vi "Parse All Elements.vi"(8 "error in":errorcluster, 11 "Node in":refnum<k20>) -> (0 "error out":errorcluster, 1 "Properties out":refnum<class "Property.lvclass">[](array[class]), 2 "Channel Data":T1, 3 "Node out":refnum<k20>)   [LabVIEW 2024, in "Parser.lvlib" / "Channel.lvclass"]
uses:
  Channel.lvclass
  Property/Property.lvclass
  <vilib>/xml/Close Reference(Node).vi
  Channel.lvclass/Channel.ctl
  <resource>/objmgr/DOMUserDefRef.rc
  <vilib>/xml/NI_XML.lvlib
  Parser.lvlib
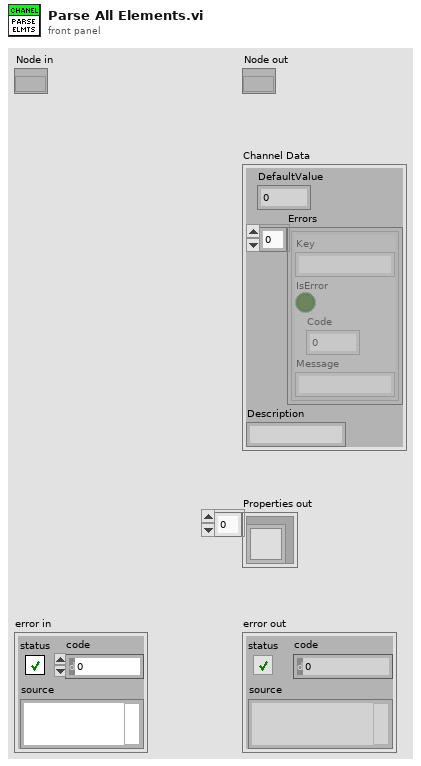
[diagram p1: front panel]
types:
  T1 = cluster{"DefaultValue":dbl, "Errors":cluster{"Key":string, "IsError":bool, "Code":u32, "Message":string}[], "Description":string}
  T2 = cluster{"Key":string, "IsError":bool, "Code":u32, "Message":string}[]
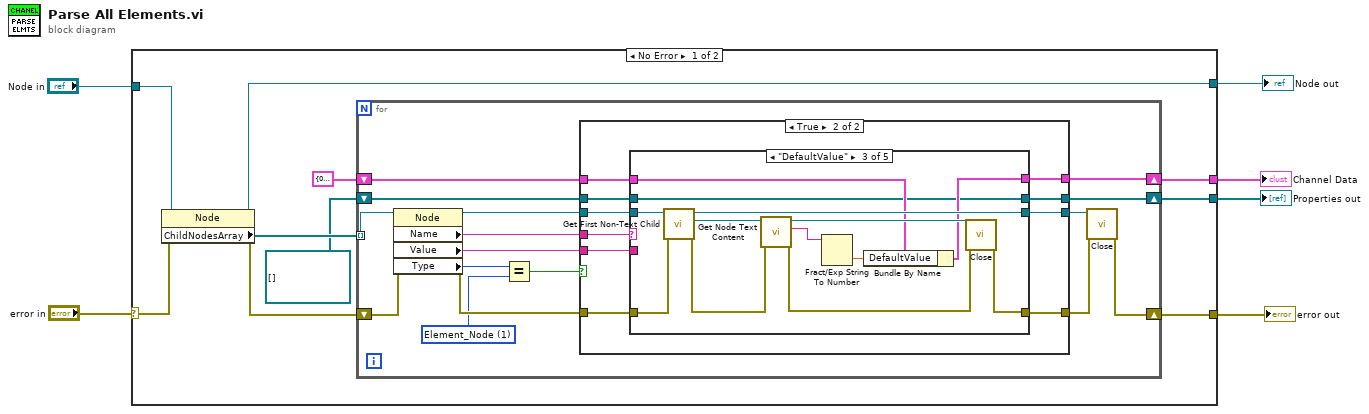
[diagram p0: block diagram]
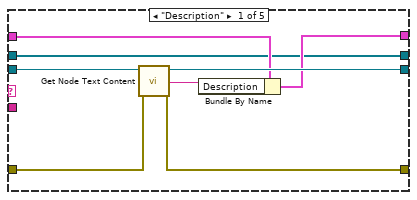
[diagram p3: hidden frame]
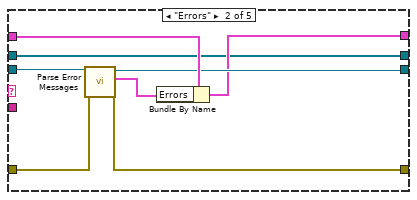
[diagram p4: hidden frame]
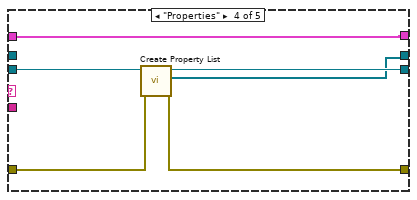
[diagram p5: hidden frame]
diagram:
  n1 = case shown="No Error" "error in" {
    selector: "error in" -> [w14 w87]
    tunnel: [w15 w87] -> w6
    tunnel: "Node in" -> [w13 w86]
    tunnel: [w11 _] -> w3
    tunnel: [w8 _] -> w2
    tunnel: [w7 w86] -> w1
    frame No Error {
      n2 = property class="Node"(reference=w13, error in=w14) -> (reference out=w7:refnum<k20>, error out=w16:errorcluster, "ChildNodesArray"=w10:refnum<k20>[])
      n3 = for {
        tunnel: w10 -> [w17] mode=indexing
        shift-right: [w31] -> w15
        shift-left: w16 -> [w32]
        shift-right: [w20] -> w11
        shift-left: T1 {"DefaultValue"=0.0, "Errors"=[], "Description"=""} ("Cluster of class private data") -> [w21]
        shift-right: [w18] -> w8
        shift-left: refnum<class "Property.lvclass">[] [] ("Properties") -> [w19]
        w24 = 1 items=["Element_Node"=1, "Attribute_Node"=2, "Text_Node"=3, "CDATASection_Node"=4, "EntityReference_Node"=5, "Entity_Node"=6, "ProcessingInstruction_Node"=7, "Comment_Node"=8, "Document_Node"=9, "DocumentType_Node"=10, "DocumentFragment_Node"=11, "Notation_Node"=12] ("Node Type")
        n4 = property on="Property Node" class="Node"(reference=w17, error in=w32) -> (reference out=w27:refnum<k20>, error out=w30:errorcluster, "Name"=w28:string, "Value"=w26:string, "Type"=w22:i32)
        n5 = Equal?(x=w22, y=w24) -> (x = y?=w23:bool)
        n6 = case shown="True" w23 {
          tunnel: w28 -> [_ w44]
          tunnel: w27 -> [w35 w43]
          tunnel: w26 -> [_ w42]
          tunnel: [w35 w41] -> w25
          tunnel: w30 -> [w36 w46]
          tunnel: [w36 w45] -> w29
          tunnel: w21 -> [w34 w40]
          tunnel: [w34 w39] -> w20
          tunnel: w19 -> [w33 w38]
          tunnel: [w33 w37] -> w18
          frame False {
          }
          frame True {
            n7 = case shown="\"DefaultValue\"" w44 {
              tunnel: w43 -> [w52 w59 w71 w79 w84]
              tunnel: w42 -> [_ _ _ _ _]
              tunnel: [w51 w58 w68 w78 w84] -> w41
              tunnel: w46 -> [w54 w62 w73 w81 w85]
              tunnel: [w53 w61 w72 w80 w85] -> w45
              tunnel: w40 -> [w49 w60 w65 w77 w83]
              tunnel: [w48 w56 w64 w77 w83] -> w39
              tunnel: w38 -> [w47 w55 w63 _ w82]
              tunnel: [w47 w55 w63 w76 w82] -> w37
              frame "Description" {
                n8 = call <vilib>:"Get Node Text Content.vi"("error in (no error)"=w54, "node in"=w52) -> ("error out"=w53:errorcluster, "node text"=w50:string, "node out"=w51:refnum<k20>)  [unwired: 7 in]
                n9 = Bundle By Name(cluster=w49, "Description"=w50) -> (w48:T1)
              }
              frame "Errors" {
                n10 = call "Parse Error Messages.vi"("error in"=w62, "Node in"=w59) -> ("error out"=w61:errorcluster, "Errors"=w57:T2, "Node out"=w58:refnum<k20>)  [unwired: 7 in]
                n11 = Bundle By Name(cluster=w60, "Errors"=w57) -> (w56:T1)
              }
              frame "DefaultValue" {
                n12 = call <vilib>:"Get First Non-Text Child.vi"("error in (no error)"=w73, "node in"=w71) -> ("error out"=w75:errorcluster, "child node"=w70:refnum<k20>, "node out"=w68:refnum<k20>)  [unwired: 6 in, 1 out]
                n13 = call <vilib>:"Get Node Text Content.vi"("error in (no error)"=w75, "node in"=w70) -> ("error out"=w74:errorcluster, "node text"=w67:string, "node out"=w69:refnum<k20>)  [unwired: 7 in]
                n14 = Fract/Exp String To Number(string=w67) -> (number=w66:dbl)  [unwired: 3 in, 1 out]
                n15 = Bundle By Name(cluster=w65, "DefaultValue"=w66) -> (w64:T1)
                n16 = call-poly <vilib>:"Close.vi"("error in (no error)"=w74, "node"=w69) -> ("error out"=w72:errorcluster)  [unwired: 7 in]
              }
              frame "Properties" {
                n17 = call "Create Property List.vi"("error in"=w81, "Property Nodes In"=w79) -> ("error out"=w80:errorcluster, "Properties out"=w76:refnum<class "Property.lvclass">[], "Property Nodes out"=w78:refnum<k20>)  [unwired: 7 in]
              }
              frame "-1", Default {
              }
            }
          }
        }
        n18 = call-poly <vilib>:"Close.vi"("error in (no error)"=w29, "node"=w25) -> ("error out"=w31:errorcluster)  [unwired: 7 in]
      }
    }
    frame Error {
    }
  }
  "error out" <- w6
  "Channel Data" <- w3
  "Properties out" <- w2
  "Node out" <- w1
